vi "ProcessName.vi"() -> (1 "process name":string)   [LabVIEW 2017, in "BlinkProcess.lvlib"]
uses:
  <vilib>/addons/BlinkProcess/BlinkProcess.lvlib
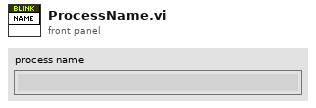
[diagram p1: front panel]
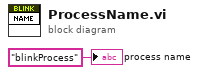
[diagram p0: block diagram]
diagram:
  "process name" <- "blinkProcess" ("ProcessName")
